vi "Bernoulli Inverse CDF.vi"(9 "p":dbl=0.2, 11 "cdf(x)":dbl=0.8) -> (0 "error":i32, 3 "x":i32)   [LabVIEW 2010, in "NI_Gmath.lvlib"]
doc: "Computes the discrete inverse cumulative distribution function (CDF), or the value <B>x</B> such that the probability that the random variate X, where X describes the selected distribution type, takes on a value less than or equal to it is <B>cdf(x)</B>. You must manually select the polymorphic instance to use."
uses:
  NI_Gmath.lvlib
  st_error_code.ctl
panel:
  # "Bernoulli Inverse CDF"
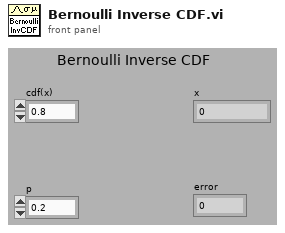
[diagram p1: front panel]
types:
  T1 = typedef "NI_Gmath.lvlib/st_error_code.ctl" = i32
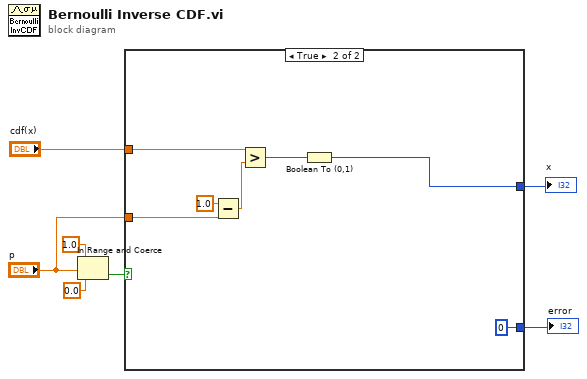
[diagram p0: block diagram]
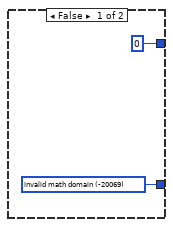
[diagram p2: hidden frame]
diagram:
  n1 = In Range and Coerce(upper limit=1.0, x="p", lower limit=0.0) -> (In Range?=w5:bool)  [unwired: 1 out]
  n2 = case shown="True" w5 {
    tunnel: [w8 0 ("invalid math domain")] -> w4
    tunnel: "p" -> [_ w14]
    tunnel: "cdf(x)" -> [_ w13]
    tunnel: [0 w10] -> w3
    frame False {
      w8 = T1 -20069 items=["invalid math domain"=-20069, "Fourier interpolation size m >= n"=-20070, "empty array"=-20003] ("stat interp error code")
    }
    frame True {
      n3 = Subtract(x=1.0, y=w14) -> (x-y=w12:dbl)
      n4 = Greater?(x=w13, y=w12) -> (0:w11:bool)
      n5 = Boolean To (0,1)(Boolean=w11) -> (0, 1=w10:i16)
    }
  }
  "x" <- w3
  "error" <- w4
